vi "Start Test.vi"(8 "ErrorIn":errorcluster, 11 "VISAIn":refnum<visa-resource-name>) -> (0 "ErrorOut":errorcluster, 2 "Data":string, 3 "VISAOut":refnum<visa-resource-name>)   [LabVIEW 2017, in "I28Drivers.lvlib"]
uses:
  I28Drivers.lvlib
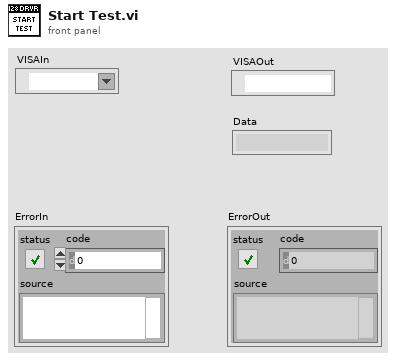
[diagram p1: front panel]
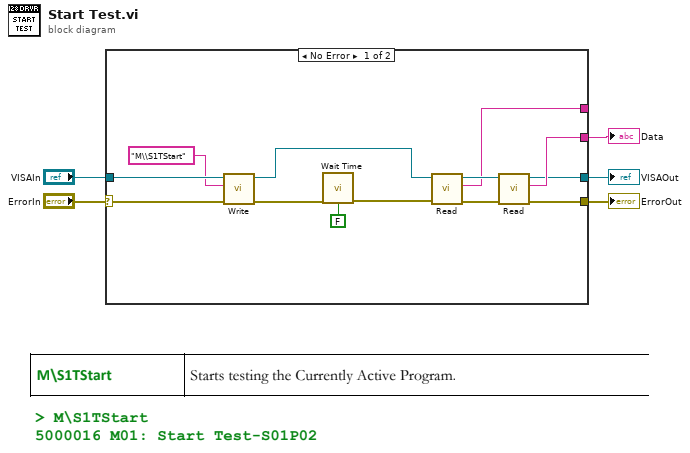
[diagram p0: block diagram]
diagram:
  n1 = case shown="No Error" "ErrorIn" {
    selector: "ErrorIn" -> [w18 w19]
    tunnel: "VISAIn" -> [w17 w20]
    tunnel: [w15 _] -> w3
    tunnel: [w14 w20] -> w1
    tunnel: [w13 w19] -> w2
    tunnel: [w10 _] -> _
    frame No Error {
      n2 = call "Write.vi"("ErrorIn"=w18, "Command"="M\\S1TStart", "VISAIn"=w17) -> ("ErrorOut"=w8:errorcluster, "VISAOut"=w9:refnum<visa-resource-name>)  [unwired: 7 in]
      n3 = call "Wait Time.vi"("error in"=w8, "Set Time"=FALSE) -> ("error out"=w7:errorcluster)  [unwired: 13 in]
      n4 = call "Read.vi"("ErrorIn"=w7, "VISAIn"=w9) -> ("ErrorOut"=w12:errorcluster, "Data"=w10:string, "VISAOut"=w11:refnum<visa-resource-name>)  [unwired: 7 in]
      n5 = call "Read.vi"("ErrorIn"=w12, "VISAIn"=w11) -> ("ErrorOut"=w13:errorcluster, "Data"=w15:string, "VISAOut"=w14:refnum<visa-resource-name>)  [unwired: 7 in]
    }
    frame Error {
    }
  }
  "ErrorOut" <- w2
  "Data" <- w3
  "VISAOut" <- w1
